vi "RSZVB Set Time Out.vi"(8 "error in (no error)":errorcluster {"code" format="%.0x"}, 10 "Timeout (10000 ms)":i32=10000, 11 "VISA session":refnum<visa-resource-name>) -> (0 "error out":errorcluster {"code" format="%.0x"}, 3 "dup VISA session":refnum<visa-resource-name>)   [LabVIEW 2011]
doc: "Sets a minimum timeout value for driver I/O transactions in milliseconds. The timeout period may vary on computer platforms."
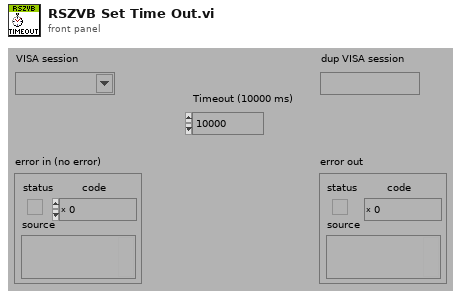
[diagram p1: front panel]
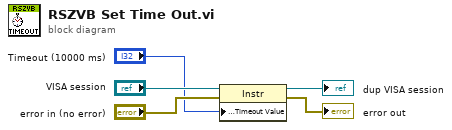
[diagram p0: block diagram]
diagram:
  n1 = property class="Instr"(reference="VISA session", error in="error in (no error)", "General Settings:Timeout Value"="Timeout (10000 ms)") -> (reference out=→"dup VISA session":refnum<visa-resource-name>, error out=→"error out":errorcluster)
